vi "ucgenalan.vi"() -> ()   [LabVIEW 2024]
panel:
  out "Numeric 4":dbl
  in  "Numeric 3":dbl
  in  "Numeric 2":dbl
  in  "Numeric":dbl
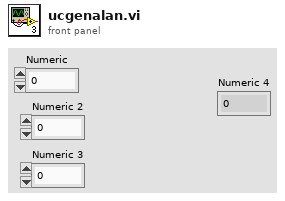
[diagram p1: front panel]
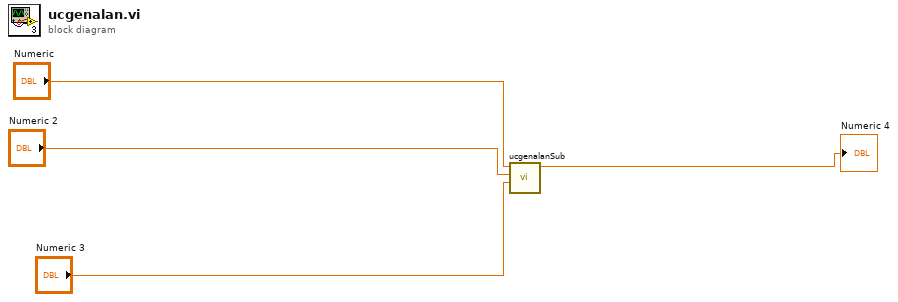
[diagram p0: block diagram]
diagram:
  n1 = call "ucgenalanSub.vi"("Numeric 3"="Numeric 3", "Numeric 2"="Numeric 2", "Numeric"="Numeric") -> ("Numeric 4"=→"Numeric 4":dbl)  [unwired: 8 in]
